vi "Result.Attributes plus Numeric into Results Table.vi"(6 "Meas":T1[](array[typedef]) {"Status" items=["LOG", "PASS", "FAIL", "ERROR"]}, 7 "File Data Objs":T3[](array[typedef]), 8 "Show Only Failures":bool, 9 "Filter":string, 10 "Attribute Data":T7[](array[typedef]) {"Status" items=["LOG", "PASS", "FAIL", "ERROR"]}, 11 "Numeric Data":T5[](array[typedef]) {"Status" items=["LOG", "PASS", "FAIL", "ERROR"]}) -> (3 "Results Table":T4[](array[typedef]))   [LabVIEW 2018]
uses:
  Result.Attribute.ctl
  Result.Measurement and Attribute Item Status.ctl
  Result.Numeric.ctl
  Result.Limit Type.ctl
  Result.Results Table Record.ctl
  Reports/Report.Result FileDataObject.ctl
  Result.Measurement Item.ctl
panel:
  in  "N/A Filler":string="n/a"
  in  "Precision (3)":i16=3
  # "Step                          Name                                             Value                      Units    LimType       LL           UL          Result        Code                     Description"
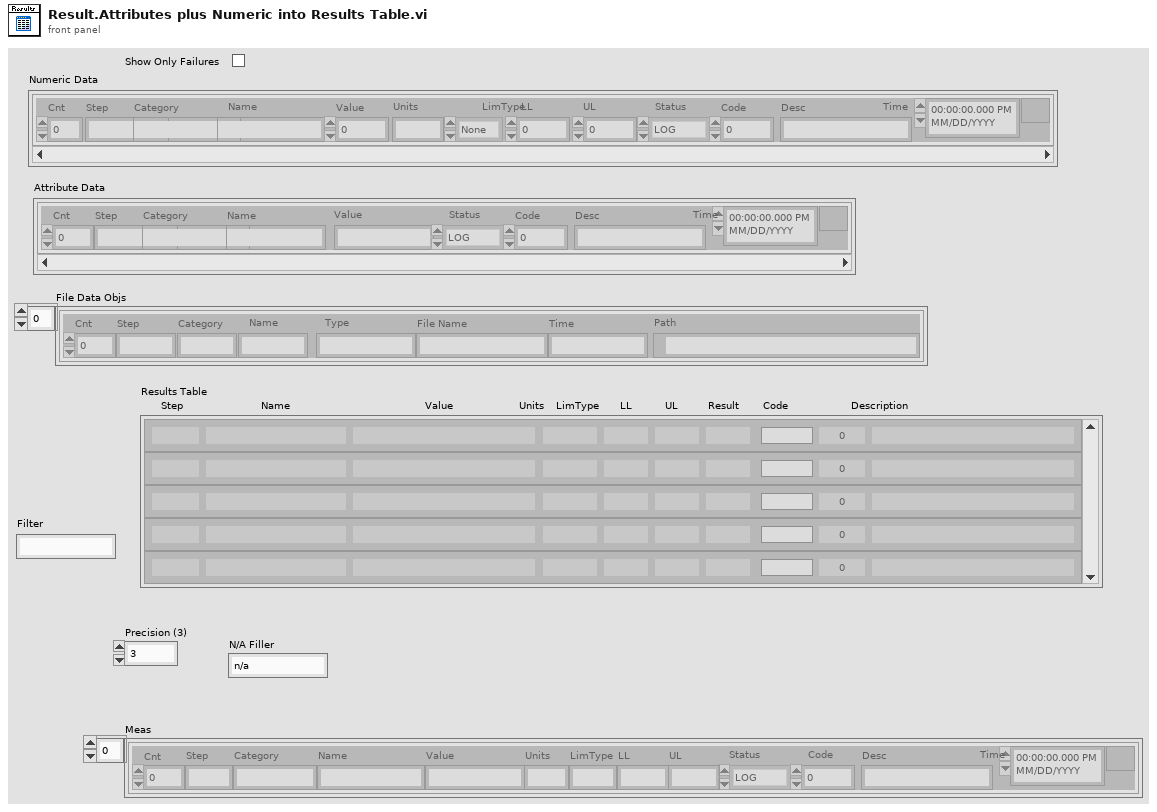
[diagram p1: front panel]
types:
  T1 = typedef "Result.Measurement Item.ctl" = cluster{"Cnt":i32, "Step":string, "Category":string, "Name":string, "Value":string, "Units":string, "LimType":string, "LL":string, "UL":string, "Status":T2, "Code":i32, "Desc":string, "Time":timestamp}
  T2 = typedef "Result.Measurement and Attribute Item Status.ctl" = i32
  T3 = typedef "Report.Result FileDataObject.ctl" = cluster{"Cnt":i32, "Step":string, "Category":string, "Name":string, "Type":string, "File Name":string, "Time":string, "Path":path}
  T4 = typedef "Result.Results Table Record.ctl" = cluster{"Cnt":i32, "Step":string, "Category":string, "Name":string, "Value":string, "Units":string, "LimType":string, "LL":string, "UL":string, "Status":string, "Status Color":u32, "Code":i32, "Desc":string}
  T5 = typedef "Result.Numeric.ctl" = cluster{"Cnt":i32, "Step":string, "Category":string, "Name":string, "Value":dbl, "Units":string, "LimType":T6, "LL":dbl, "UL":dbl, "Status":T2, "Code":i32, "Desc":string, "Time":timestamp}
  T6 = typedef "Result.Limit Type.ctl" = enum16{"None", "EQ", "NE", "GT", "LT", "GE", "LE", "GTLT", "GELE", "GELT", "GTLE", "LTGT", "LEGE", "LEGT", "LTGE", "Contains", "NotContains"}
  T7 = typedef "Result.Attribute.ctl" = cluster{"Cnt":i32, "Step":string, "Category":string, "Name":string, "Value":string, "Status":T2, "Code":i32, "Desc":string, "Time":timestamp}
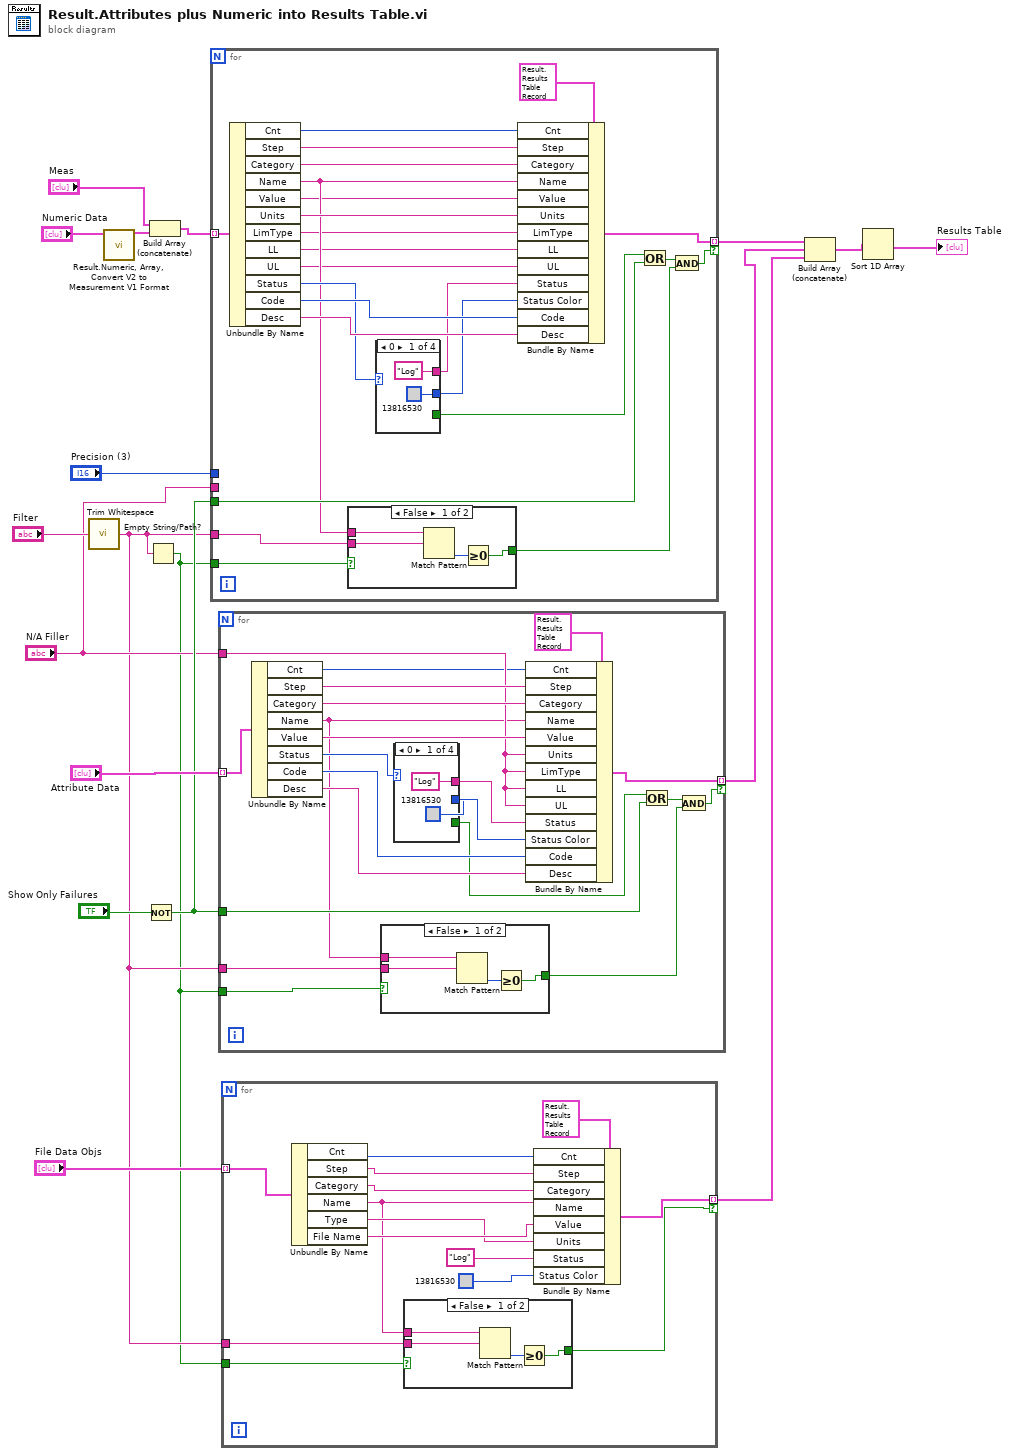
[diagram p0: block diagram]
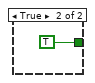
[diagram p2: hidden frame]
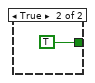
[diagram p3: hidden frame]
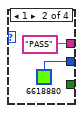
[diagram p4: hidden frame]
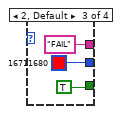
[diagram p5: hidden frame]
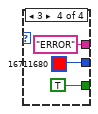
[diagram p6: hidden frame]
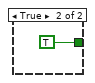
[diagram p7: hidden frame]
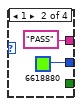
[diagram p8: hidden frame]
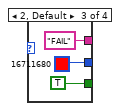
[diagram p9: hidden frame]
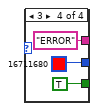
[diagram p10: hidden frame]
diagram:
  n1 = call <vilib>:"Trim Whitespace.vi"("string"="Filter") -> ("trimmed string"=w6:string)  [unwired: 1 in]
  n2 = call "Result.Numeric, Array, Convert V2 to Measurement V1 Format.vi"("Num In"="Numeric Data") -> ("Meas Out"=w3:T1[])  [unwired: 10 in]
  n3 = Not(x="Show Only Failures") -> (.not. x?=w11:bool)
  n4 = Empty String/Path?(string/path=w6) -> (empty?=w5:bool)
  n5 = Build Array (concatenate)("Meas", w3) -> (w1:T1[])
  n6 = for {
    tunnel: w1 -> [w41] mode=indexing
    tunnel: "Precision (3)" -> [_]
    tunnel: [w35] -> w17 mode=indexing if=w25
    tunnel: w11 -> [w29]
    tunnel: w6 -> [w27]
    tunnel: w5 -> [w23]
    tunnel: "N/A Filler" -> [_]
    n7 = Unbundle By Name(w41) -> ("Cnt"=w31:i32, "Step"=w40:string, "Category"=w39:string, "Name"=w28:string, "Value"=w22:string, "Units"=w36:string, "LimType"=w21:string, "LL"=w20:string, "UL"=w19:string, "Status"=w34:T2, "Code"=w37:i32, "Desc"=w38:string)
    n8 = case shown="False" w23 {
      tunnel: w27 -> [w46 _]
      tunnel: w28 -> [w45 _]
      tunnel: [w43 TRUE] -> w24
      frame False {
        n9 = Match Pattern(string=w45, regular expression=w46) -> (offset past match=w44:i32)  [unwired: 1 in, 3 out]
        n10 = Greater Or Equal To 0?(x=w44) -> (x >= 0?=w43:bool)
      }
      frame True {
      }
    }
    n11 = case shown="0" w34 {
      tunnel: [u32 13816530 u32 6618880 u32 16711680 u32 16711680] -> w32
      tunnel: ["Log" "PASS" "FAIL" "ERROR"] -> w33
      tunnel: [_ _ TRUE TRUE] -> w30
      frame 0 {
      }
      frame 1 {
      }
      frame 2, Default {
      }
      frame 3 {
      }
    }
    n12 = Bundle By Name(cluster=T4 {"Cnt"=0, "Step"="", "Category"="", "Name"="", "Value"="", "Units"="", "LimType"="", "LL"="", "UL"="", "Status"="", "Status Color"=16448250, "Code"=0, "Desc"=""} ("Results Table Record"), "Cnt"=w31, "Step"=w40, "Category"=w39, "Name"=w28, "Value"=w22, "Units"=w36, "LimType"=w21, "LL"=w20, "UL"=w19, "Status"=w33, "Status Color"=w32, "Code"=w37, "Desc"=w38) -> (w35:T4)
    n13 = Or(x=w30, y=w29) -> (x .or. y?=w26:bool)
    n14 = And(x=w26, y=w24) -> (x .and. y?=w25:bool)
  }
  n15 = for {
    tunnel: "Attribute Data" -> [w77] mode=indexing
    tunnel: [w72] -> w16 mode=indexing if=w62
    tunnel: "N/A Filler" -> [w68]
    tunnel: w11 -> [w65]
    tunnel: w6 -> [w59]
    tunnel: w5 -> [w58]
    n16 = Unbundle By Name(w77) -> ("Cnt"=w66:i32, "Step"=w76:string, "Category"=w75:string, "Name"=w60:string, "Value"=w69:string, "Status"=w71:T2, "Code"=w73:i32, "Desc"=w74:string)
    n17 = case shown="False" w58 {
      tunnel: w59 -> [w82 _]
      tunnel: w60 -> [w81 _]
      tunnel: [w79 TRUE] -> w61
      frame False {
        n18 = Match Pattern(string=w81, regular expression=w82) -> (offset past match=w80:i32)  [unwired: 1 in, 3 out]
        n19 = Greater Or Equal To 0?(x=w80) -> (x >= 0?=w79:bool)
      }
      frame True {
      }
    }
    n20 = case shown="0" w71 {
      tunnel: [u32 13816530 u32 6618880 u32 16711680 u32 16711680] -> w70
      tunnel: ["Log" "PASS" "FAIL" "ERROR"] -> w67
      tunnel: [_ _ TRUE TRUE] -> w64
      frame 0 {
      }
      frame 1 {
      }
      frame 2, Default {
      }
      frame 3 {
      }
    }
    n21 = Bundle By Name(cluster=T4 {"Cnt"=0, "Step"="", "Category"="", "Name"="", "Value"="", "Units"="", "LimType"="", "LL"="", "UL"="", "Status"="", "Status Color"=16448250, "Code"=0, "Desc"=""} ("Results Table Record"), "Cnt"=w66, "Step"=w76, "Category"=w75, "Name"=w60, "Value"=w69, "Units"=w68, "LimType"=w68, "LL"=w68, "UL"=w68, "Status"=w67, "Status Color"=w70, "Code"=w73, "Desc"=w74) -> (w72:T4)
    n22 = Or(x=w64, y=w65) -> (x .or. y?=w63:bool)
    n23 = And(x=w63, y=w61) -> (x .and. y?=w62:bool)
  }
  n24 = for {
    tunnel: "File Data Objs" -> [w106] mode=indexing
    tunnel: [w100] -> w7 mode=indexing if=w96
    tunnel: w6 -> [w98]
    tunnel: w5 -> [w97]
    n25 = Unbundle By Name(w106) -> ("Cnt"=w105:i32, "Step"=w104:string, "Category"=w103:string, "Name"=w99:string, "Type"=w101:string, "File Name"=w102:string)
    n26 = case shown="False" w97 {
      tunnel: w98 -> [w111 _]
      tunnel: w99 -> [w110 _]
      tunnel: [w108 TRUE] -> w96
      frame False {
        n27 = Match Pattern(string=w110, regular expression=w111) -> (offset past match=w109:i32)  [unwired: 1 in, 3 out]
        n28 = Greater Or Equal To 0?(x=w109) -> (x >= 0?=w108:bool)
      }
      frame True {
      }
    }
    n29 = Bundle By Name(cluster=T4 {"Cnt"=0, "Step"="", "Category"="", "Name"="", "Value"="", "Units"="", "LimType"="", "LL"="", "UL"="", "Status"="", "Status Color"=16448250, "Code"=0, "Desc"=""} ("Results Table Record"), "Cnt"=w105, "Step"=w104, "Category"=w103, "Name"=w99, "Value"=w102, "Units"=w101, "Status"="Log", "Status Color"=u32 13816530) -> (w100:T4)
  }
  n30 = Build Array (concatenate)(w17, w16, w7) -> (w14:T4[])
  n31 = Sort 1D Array(array=w14) -> (sorted array=→"Results Table":T4[])
